vi "Get Output Values.vi"(8 "error in (no error)":errorcluster, 10 "Number of points":i32, 11 "Spectrum Recorder in":refnum<class "Spectrum Recorder.lvclass">) -> (0 "error out":errorcluster, 2 "Output values":dbl[](array[numeric]), 3 "Spectrum Recorder out":refnum<class "Spectrum Recorder.lvclass">)   [LabVIEW 2016, in "Spectrum Recorder.lvclass"]
uses:
  Spectrum Recorder.lvclass
  Spectrum Recorder.lvclass/Spectrum Recorder.ctl
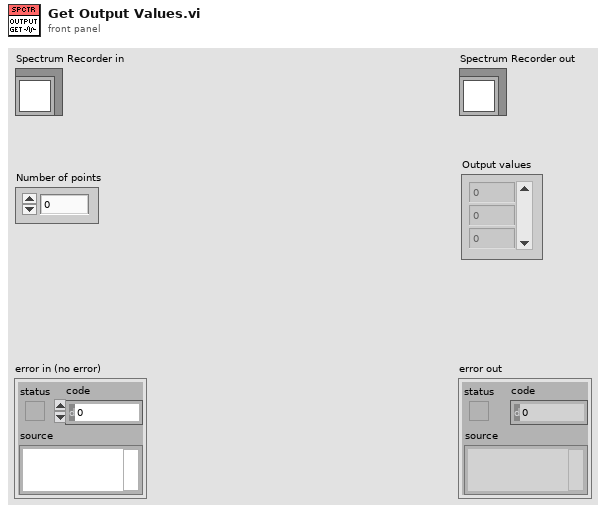
[diagram p1: front panel]
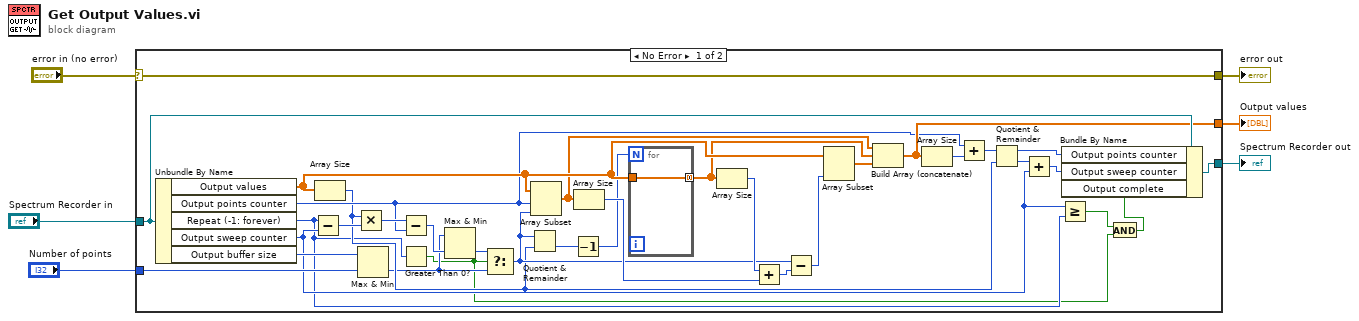
[diagram p0: block diagram]
diagram:
  n1 = case shown="No Error" "error in (no error)" {
    selector: "error in (no error)" -> [w40 w43]
    tunnel: [w40 w43] -> w5
    tunnel: [w30 w42] -> w3
    tunnel: "Spectrum Recorder in" -> [w39 w42]
    tunnel: "Number of points" -> [w13 _]
    tunnel: [w21 _] -> w1
    frame No Error {
      n2 = Unbundle By Name(w39) -> ("Output values"=w36:dbl[], "Output points counter"=w19:i32, "Repeat (-1: forever)"=w10:i32, "Output sweep counter"=w11:i32, "Output buffer size"=w14:i32)
      n3 = Subtract(x=w10, y=w11) -> (x-y=w38:i32)
      n4 = Array Size(array=w36) -> (size(s)=w17:i32)
      n5 = Multiply(x=w17, y=w38) -> (x*y=w28:i32)
      n6 = Max & Min(x=w14, y=w13) -> (min(x,y)=w12:i32)  [unwired: 1 out]
      n7 = Subtract(x=w28, y=w19) -> (x-y=w27:i32)
      n8 = Greater Than 0?(x=w10) -> (x > 0?=w8:bool)
      n9 = Max & Min(x=w12, y=w27) -> (min(x,y)=w25:i32)  [unwired: 1 out]
      n10 = Select(t=w25, s=w8, f=w12) -> (s? t:f=w24:i32)
      n11 = Quotient & Remainder(x=w24, y=w17) -> (floor(x/y)=w23:i32)  [unwired: 1 out]
      n12 = Array Subset(array=w36, index=w19, length=w24) -> (w34:dbl[])
      n13 = Decrement(x=w23) -> (x-1=w26:i32)
      n14 = Array Size(array=w34) -> (size(s)=w32:i32)
      n15 = for {
        N: w26 -> [_]
        tunnel: [w41] -> w35 mode=concatenating
        tunnel: w36 -> [w41]
      }
      n16 = Array Size(array=w35) -> (size(s)=w33:i32)
      n17 = Add(x=w33, y=w32) -> (x+y=w31:i32)
      n18 = Subtract(x=w24, y=w31) -> (x-y=w29:i32)
      n19 = Array Subset(array=w36, length=w29) -> (w37:dbl[])  [unwired: 1 in]
      n20 = Build Array (concatenate)(w34, w35, w37) -> (w21:dbl[])
      n21 = Array Size(array=w21) -> (size(s)=w20:i32)
      n22 = Add(x=w19, y=w20) -> (x+y=w18:i32)
      n23 = Quotient & Remainder(x=w18, y=w17) -> (x-y*floor(x/y)=w16:i32, floor(x/y)=w15:i32)
      n24 = Add(x=w15, y=w11) -> (x+y=w22:i32)
      n25 = Greater Or Equal?(x=w11, y=w10) -> (x >= y?=w9:bool)
      n26 = And(x=w9, y=w8) -> (x .and. y?=w7:bool)
      n27 = Bundle By Name(cluster=w39, "Output points counter"=w16, "Output sweep counter"=w22, "Output complete"=w7) -> (w30:refnum<class "Spectrum Recorder.lvclass">)
    }
    frame Error {
    }
  }
  "error out" <- w5
  "Spectrum Recorder out" <- w3
  "Output values" <- w1
